vi "PrelabSetup.vi"() -> ()   [LabVIEW 2018]
uses:
  <vilib>/Analysis/NI_AALBase.lvlib
panel:
  out "Waveform Graph 2":waveform(dbl)(graph)
  out "Waveform Graph":dbl[](graph)
  in  "Sample Rate(Sa/s)":dbl
  in  "Amplitude":dbl
  in  "Frequency (Hz)":dbl
  in  "Duration(sec)":dbl
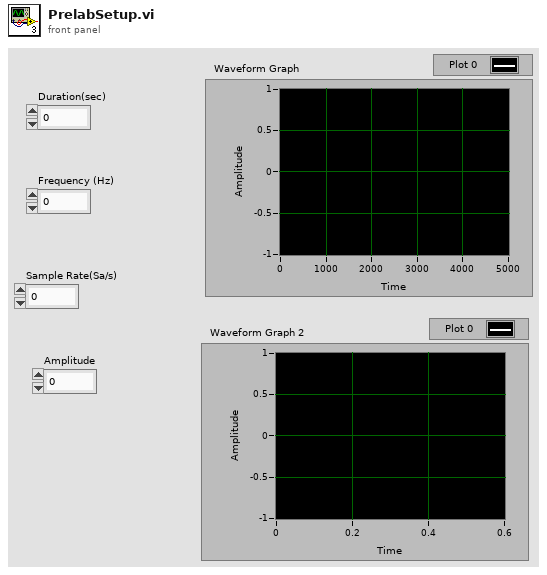
[diagram p1: front panel]
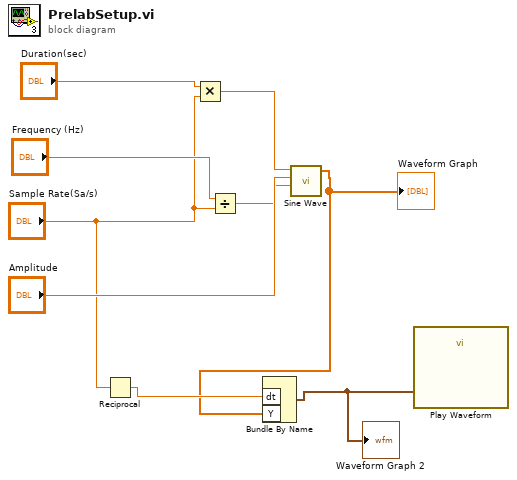
[diagram p0: block diagram]
diagram:
  n1 = Reciprocal(x="Sample Rate(Sa/s)") -> (1/x=w3:dbl)
  n2 = Multiply(x="Duration(sec)", y="Sample Rate(Sa/s)") -> (x*y=w7:dbl)
  n3 = Divide(x="Frequency (Hz)", y="Sample Rate(Sa/s)") -> (x/y=w5:dbl)
  n4 = call <vilib>:"Sine Wave.vi"("samples"=w7, "amplitude"="Amplitude", "frequency"=w5) -> ("sine wave"=w2:dbl[])  [unwired: 2 in, 2 out]
  "Waveform Graph" <- w2
  n5 = Bundle By Name("dt"=w3, "Y"=w2) -> (w1:waveform(dbl))  [unwired: 1 in]
  "Waveform Graph 2" <- w1
  n6 = call "Play Waveform"("Data"=w1) -> ()  [unwired: 18 in, 1 out]
